vi "Read commandName.vi"(8 "error in (no error)":errorcluster, 11 "OnHeartbeat in":refnum<class "OnHeartbeat.lvclass">) -> (0 "error out":errorcluster, 2 "Enum":T1(ring), 3 "OnHeartbeat out":refnum<class "OnHeartbeat.lvclass">)   [LabVIEW 2016, in "Commands.lvlib" / "OnHeartbeat.lvclass"]
uses:
  OnHeartbeat.lvclass
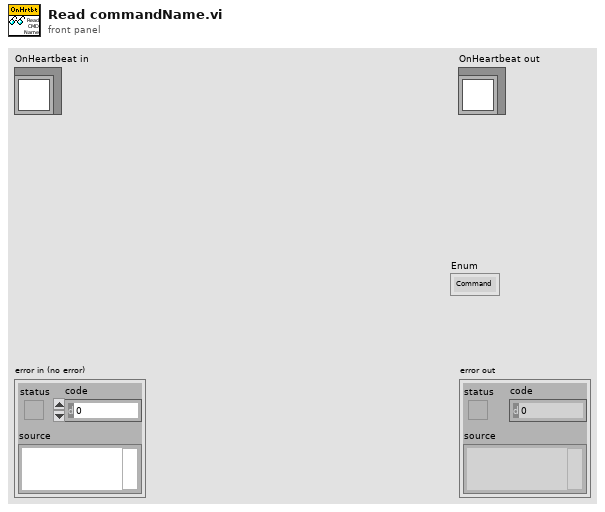
[diagram p1: front panel]
types:
  T1 = enum16{"Command", "Start", "ClearError", "HeartBeat", "Enable", "Disable", "Standby", "Exit", "OnInterrupt", "OnIncomingMessagingError"}
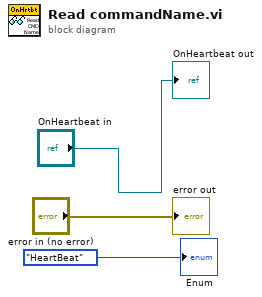
[diagram p0: block diagram]
diagram:
  "error out" <- "error in (no error)"
  "OnHeartbeat out" <- "OnHeartbeat in"
  "Enum" <- T1."HeartBeat"
